vi "Get Raw RGB.vi"(8 "Error In":errorcluster, 11 "Index":i32) -> (0 "Error Out":errorcluster, 2 "Timestamp (ms)":u32, 3 "Raw RGB Data":cluster{"Red":dbl, "Green":dbl, "Blue":dbl}[][](array[cluster]))   [LabVIEW 2011, in "LVH-Interface-for-Kinect.lvlib"]
uses:
  <vilib>/LabVIEW Hacker/LVH-Interface-for-Kinect/LVH-Interface-for-Kinect.lvlib
  <vilib>/LabVIEW Hacker/LVH-Interface-for-Kinect/Public/lib/freenect_sync.dll
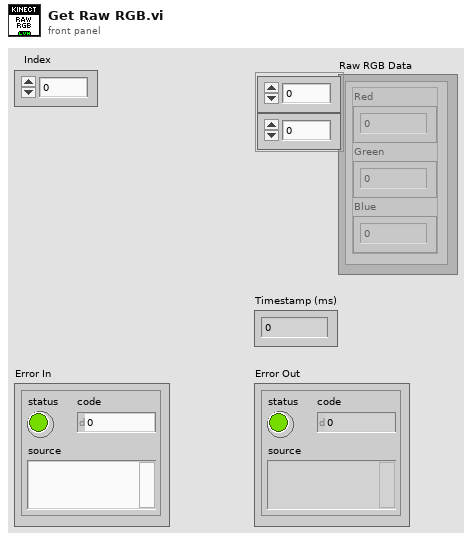
[diagram p1: front panel]
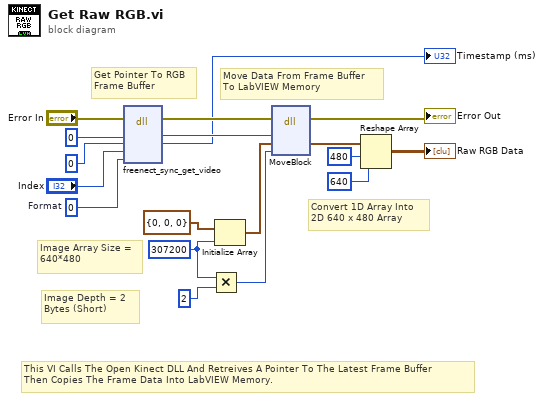
[diagram p0: block diagram]
diagram:
  w9 = u16 0  # Format
  w16 = 307200 ("dimension size")
  # "This VI Calls The Open Kinect DLL And Retreives A Pointer To The Latest Frame Buffer\nThen Copies The Frame Data Into LabVIEW Memory."
  # "Move Data From Frame Buffer\nTo LabVIEW Memory"
  # "Convert 1D Array Into \n2D 640 x 480 Array"
  # "Get Pointer To RGB\nFrame Buffer"
  # "Image Depth = 2 Bytes (Short)"
  # "Image Array Size = 640*480"
  n1 = dll-call lib="C:/Program Files (x86)/National Instruments/LabVIEW 2011/vi.lib/LabVIEW Hacker/LVH-Interface-for-Kinect/Public/lib/freenect_sync.dll" fn="freenect_sync_get_video"(error in="Error In", "ptr"=i64 0, "timestamp"=u32 0, "index"="Index", "fmt"=w9) -> (error out=w18:errorcluster, "ptr"=w13:i64, "timestamp"=→"Timestamp (ms)":u32)  [unwired: 3 in, 3 out]
  n2 = Multiply(x=w16, y=2) -> (x*y=w14:i32)
  n3 = Initialize Array(cluster{"R":u8, "G":u8, "B":u8} {"R"=0, "G"=0, "B"=0} ("RGB24bit"), w16) -> (w17:cluster{"R":u8, "G":u8, "B":u8}[])
  n4 = dll-call lib="LabVIEW" fn="MoveBlock"(error in=w18, "Address (Pointer)"=w13, "Destination"=w17, "Size"=w14) -> (error out=→"Error Out":errorcluster, "Destination"=w8:cluster{"R":u8, "G":u8, "B":u8}[])  [unwired: 4 in, 2 out]
  n5 = Reshape Array(w8, 480 ("dimension size"), 640 ("dimension size")) -> (→"Raw RGB Data":cluster{"R":u8, "G":u8, "B":u8}[][])
